vi "VL53L0X_SetVcselPulsePeriod.vi"(9 "VCSELPulsePeriodPCLK Final":u8, 10 "VCSELPulsePeriodPCLK Pre":u8, 11 "REV2mDistanceSensorDevRef":T1) -> (3 "REV2mDistanceSensorDevRef Out":T1)   [LabVIEW 2019, in "DistanceSensorDriver.lvlib"]
uses:
  DistanceSensorDriver.lvlib
  Typedef/REV2mDistanceSensorDevRef.ctl
  Typedef/Ports.ctl
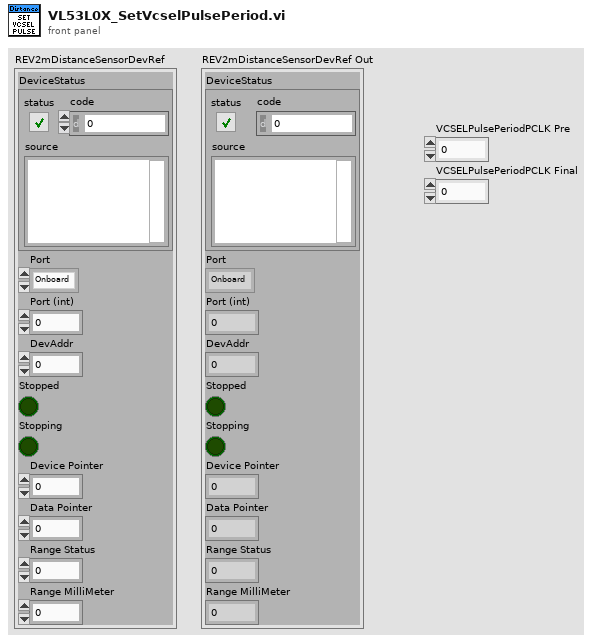
[diagram p1: front panel]
types:
  T1 = typedef "DistanceSensorDriver.lvlib/REV2mDistanceSensorDevRef.ctl" = cluster{"DeviceStatus":errorcluster, "Port":T2, "Port (int)":i32, "DevAddr":i32, "Stopped":bool, "Stopping":bool, "Device Pointer":u64, "Data Pointer":u64, "Range Status":u8, "Range MilliMeter":u16}
  T2 = typedef "DistanceSensorDriver.lvlib/Ports.ctl" = enum32{"Onboard", "MXP"}
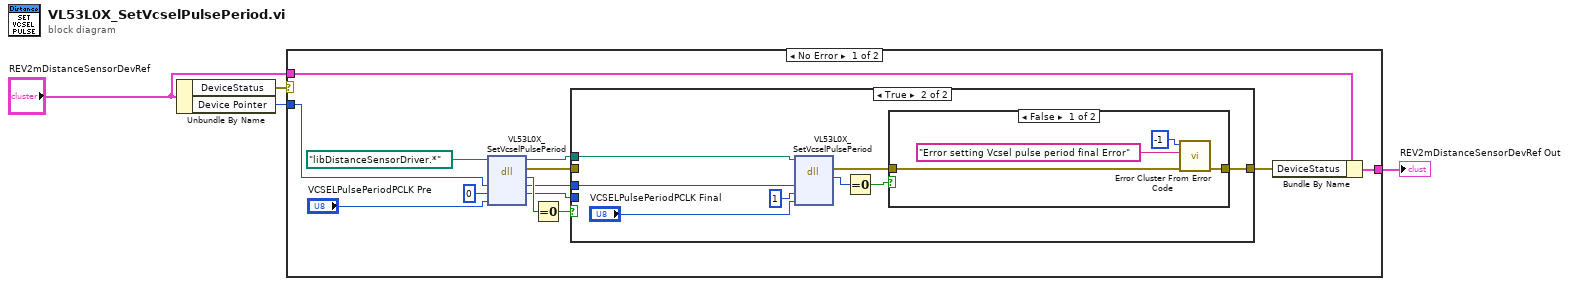
[diagram p0: block diagram]
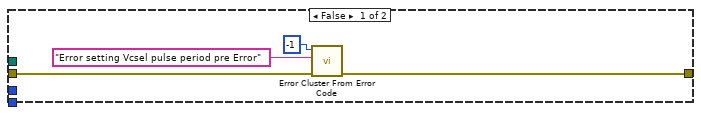
[diagram p2: hidden frame]
diagram:
  n1 = Unbundle By Name("REV2mDistanceSensorDevRef") -> ("DeviceStatus"=w1:errorcluster, "Device Pointer"=w4:u64)
  n2 = case shown="No Error" w1 {
    tunnel: w4 -> [w12 _]
    tunnel: [w11 w35] -> w3
    tunnel: "REV2mDistanceSensorDevRef" -> [w10 w35]
    frame No Error {
      n3 = dll-call lib="?" fn="VL53L0X_SetVcselPulsePeriod"(path in=path "libDistanceSensorDriver.*", "Dev"=w12, "VcselPeriodType"=u8 0, "VCSELPulsePeriodPCLK"="VCSELPulsePeriodPCLK Pre") -> (path out=w7:path, error out=w13:errorcluster, "Status"=w14:i32, "Dev"=w9:u64, "VcselPeriodType"=w8:u8)  [unwired: 3 in]
      n4 = Equal To 0?(x=w14) -> (x = 0?=w17:bool)
      n5 = case shown="True" w17 {
        tunnel: w13 -> [w18 _]
        tunnel: [w21 w28] -> w16
        tunnel: w9 -> [_ w25]
        tunnel: w8 -> [_ _]
        tunnel: w7 -> [_ w26]
        frame False {
          n6 = call <vilib>:"Error Cluster From Error Code.vi"("error in (no error)"=w18, "error message (\"\")"="Error setting Vcsel pulse period pre Error" ("error message (\"\")"), "error code (0)"=-1) -> ("error out"=w21:errorcluster)  [unwired: 6 in]
        }
        frame True {
          n7 = dll-call lib="?" fn="VL53L0X_SetVcselPulsePeriod"(path in=w26, "Dev"=w25, "VcselPeriodType"=u8 1, "VCSELPulsePeriodPCLK"="VCSELPulsePeriodPCLK Final") -> (error out=w27:errorcluster, "Status"=w24:i32)  [unwired: 5 in, 1 out]
          n8 = Equal To 0?(x=w24) -> (x = 0?=w29:bool)
          n9 = case shown="False" w29 {
            tunnel: w27 -> [w31 w34]
            tunnel: [w30 w34] -> w28
            frame False {
              n10 = call <vilib>:"Error Cluster From Error Code.vi"("error in (no error)"=w31, "error message (\"\")"="Error setting Vcsel pulse period final Error" ("error message (\"\")"), "error code (0)"=-1) -> ("error out"=w30:errorcluster)  [unwired: 6 in]
            }
            frame True {
            }
          }
        }
      }
      n11 = Bundle By Name(cluster=w10, "DeviceStatus"=w16) -> (w11:T1)
    }
    frame Error {
    }
  }
  "REV2mDistanceSensorDevRef Out" <- w3
